vi "niRFUtil CONV 1 Ohm Voltage to dBm (complex wfm).vi"(2 "Reduced Precision?":bool, 7 "Complex Waveform (V)":T3 {"y" format="%.2f"; "dx" format="%^.2e"; "x0" format="%^.2e"}) -> (8 "Real Waveform (dBm)":T1 {"y" min=0 max=127 format="%.2f"; "dx" format="%^.2e"; "x0" format="%^.2e"})   [LabVIEW 2015, in "niRFUtil.lvlib"]
doc: "(c) Copyright 2006, National Instruments, Inc. This VI may not be duplicated, sold, or distributed without written consent from National Instruments."
uses:
  niRFUtil.lvlib
  Includes/niRFUtil INC Complex Waveform.ctl
  Includes/niRFUtil INC Complex Array.ctl
  Includes/niRFUtil INC Real Waveform.ctl
  Includes/niRFUtil INC Real Array.ctl
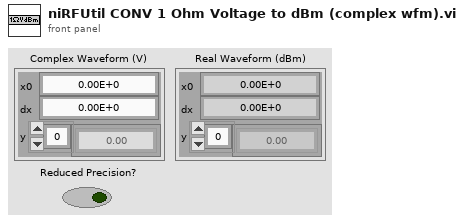
[diagram p1: front panel]
types:
  T1 = typedef "niRFUtil.lvlib/niRFUtil INC Real Waveform.ctl" = cluster{"x0":dbl, "dx":dbl, "y":T2}
  T2 = typedef "niRFUtil.lvlib/niRFUtil INC Real Array.ctl" = sgl[]
  T3 = typedef "niRFUtil.lvlib/niRFUtil INC Complex Waveform.ctl" = cluster{"x0":dbl, "dx":dbl, "y":T4}
  T4 = typedef "niRFUtil.lvlib/niRFUtil INC Complex Array.ctl" = csg[]
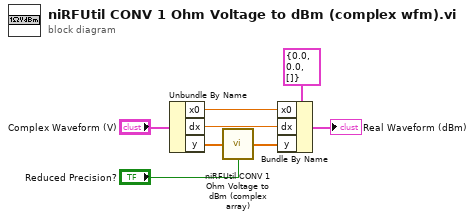
[diagram p0: block diagram]
diagram:
  n1 = Unbundle By Name("Complex Waveform (V)") -> ("x0"=w5:dbl, "dx"=w4:dbl, "y"=w3:T4)
  n2 = call "niRFUtil CONV 1 Ohm Voltage to dBm (complex array).vi"("Reduced Precision?"="Reduced Precision?", "Complex Array (V)"=w3) -> ("Real Array (dBm)"=w2:T2)  [unwired: 13 in]
  n3 = Bundle By Name(cluster=T1 {"x0"=0.0, "dx"=0.0, "y"=[]} ("Real Waveform (dBm)"), "x0"=w5, "dx"=w4, "y"=w2) -> (→"Real Waveform (dBm)":T1)
